vi "svc_Convert Frequency to Frequency String.vi"(7 "number of decimal places to add":i32, 10 "x-axis unit label":string="Hz", 11 "frequency [Hz]":dbl format="%.2f") -> (3 "frequency string":string)   [LabVIEW 2017]
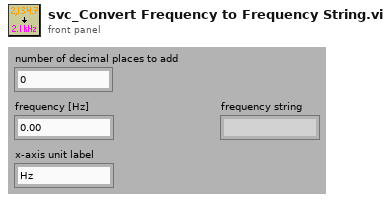
[diagram p1: front panel]
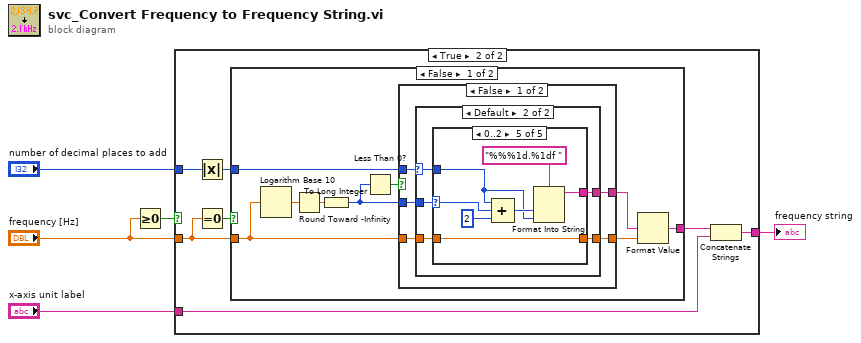
[diagram p0: block diagram]
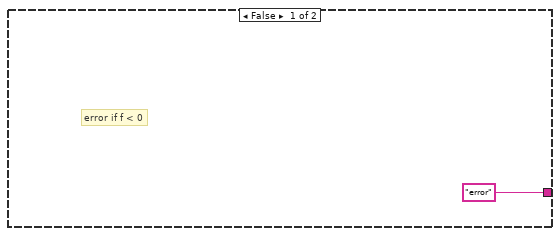
[diagram p2: hidden frame]
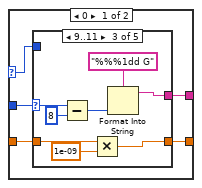
[diagram p3: hidden frame]
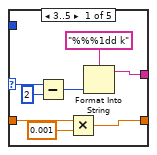
[diagram p4: hidden frame]
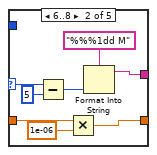
[diagram p5: hidden frame]
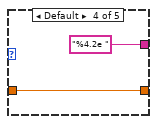
[diagram p6: hidden frame]
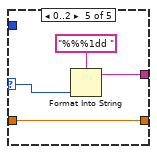
[diagram p7: hidden frame]
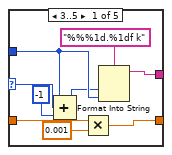
[diagram p8: hidden frame]
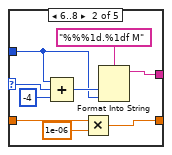
[diagram p9: hidden frame]
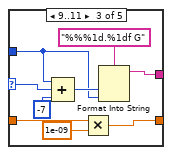
[diagram p10: hidden frame]
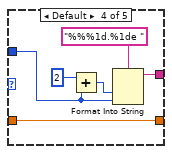
[diagram p11: hidden frame]
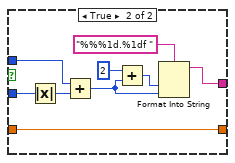
[diagram p12: hidden frame]
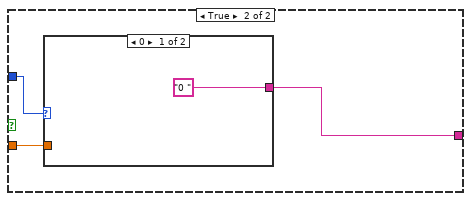
[diagram p13: hidden frame]
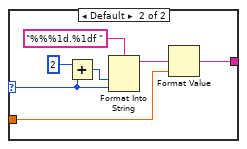
[diagram p14: hidden frame]
diagram:
  n1 = Greater Or Equal To 0?(x="frequency [Hz]") -> (x >= 0?=w3:bool)
  n2 = case shown="True" w3 {
    tunnel: ["error" ("output string") w9] -> w5
    tunnel: "frequency [Hz]" -> [_ w12]
    tunnel: "number of decimal places to add" -> [_ w11]
    tunnel: "x-axis unit label" -> [_ w7]
    frame False {
      # "error if f < 0"
    }
    frame True {
      n3 = Absolute Value(x=w11) -> (abs(x)=w10:i32)
      n4 = Equal To 0?(x=w12) -> (x = 0?=w13:bool)
      n5 = case shown="False" w13 {
        tunnel: [w22 w117] -> w8
        tunnel: w12 -> [w16 w118]
        tunnel: w10 -> [w14 w119]
        frame False {
          n6 = Logarithm Base 10(1:w16) -> (0:w17:dbl)
          n7 = Round Toward -Infinity ("Round To -Infinity")(1:w17) -> (0:w21:dbl)
          n8 = To Long Integer(number=w21) -> (32bit integer=w19:i32)
          n9 = Less Than 0?(x=w19) -> (x < 0?=w20:bool)
          n10 = case shown="False" w20 {
            tunnel: w19 -> [w27 w114]
            tunnel: [w26 w112] -> w18
            tunnel: w16 -> [w25 w111]
            tunnel: [w24 w111] -> w15
            tunnel: w14 -> [w23 w109]
            frame False {
              n11 = case shown="Default" w23 {
                selector: w23 -> [w31 w63]
                tunnel: w27 -> [w32 w67]
                tunnel: [w29 w66] -> w26
                tunnel: w25 -> [w30 w65]
                tunnel: [w28 w64] -> w24
                frame 0 {
                  n12 = case shown="9..11" w32 {
                    selector: w32 -> [w36 w44 w52 _ w59]
                    tunnel: [w34 w42 w50 "%4.2e " ("format string") w60] -> w29
                    tunnel: w30 -> [w40 w48 w56 w58 w62]
                    tunnel: [w38 w46 w54 w58 w62] -> w28
                    tunnel: w31 -> [_ _ _ _ _]
                    frame 3..5 {
                      n13 = Subtract(x=w36, y=2) -> (x-y=w37:i32)
                      n14 = Multiply(x=w40, y=0.001) -> (x*y=w38:dbl)
                      n15 = Format Into String(format string="%%%1dd k", w37) -> (resulting string=w34:string)  [unwired: 2 in, 1 out]
                    }
                    frame 6..8 {
                      n16 = Subtract(x=w44, y=5) -> (x-y=w45:i32)
                      n17 = Multiply(x=w48, y=1e-06) -> (x*y=w46:dbl)
                      n18 = Format Into String(format string="%%%1dd M", w45) -> (resulting string=w42:string)  [unwired: 2 in, 1 out]
                    }
                    frame 9..11 {
                      n19 = Subtract(x=w52, y=8) -> (x-y=w53:i32)
                      n20 = Multiply(x=w56, y=1e-09) -> (x*y=w54:dbl)
                      n21 = Format Into String(format string="%%%1dd G", w53) -> (resulting string=w50:string)  [unwired: 2 in, 1 out]
                    }
                    frame Default {
                    }
                    frame 0..2 {
                      n22 = Format Into String(format string="%%%1dd ", w59) -> (resulting string=w60:string)  [unwired: 2 in, 1 out]
                    }
                  }
                }
                frame Default {
                  n23 = case shown="0..2" w67 {
                    selector: w67 -> [w71 w82 w91 _ w106]
                    tunnel: [w73 w81 w90 w97 w101] -> w66
                    tunnel: w65 -> [w76 w85 w94 w100 w107]
                    tunnel: [w74 w83 w92 w100 w107] -> w64
                    tunnel: w63 -> [w70 w79 w87 w98 w103]
                    frame 3..5 {
                      n24 = Compound Arithmetic op=ADD(w70, w71, -1 ("y")) -> (w69:i32)
                      n25 = Multiply(x=w76, y=0.001) -> (x*y=w74:dbl)
                      n26 = Format Into String(format string="%%%1d.%1df k", w69, w70) -> (resulting string=w73:string)  [unwired: 2 in, 1 out]
                    }
                    frame 6..8 {
                      n27 = Compound Arithmetic op=ADD(w79, w82, -4 ("value")) -> (w80:i32)
                      n28 = Multiply(x=w85, y=1e-06) -> (x*y=w83:dbl)
                      n29 = Format Into String(format string="%%%1d.%1df M", w80, w79) -> (resulting string=w81:string)  [unwired: 2 in, 1 out]
                    }
                    frame 9..11 {
                      n30 = Compound Arithmetic op=ADD(w87, w91, -7 ("value")) -> (w88:i32)
                      n31 = Multiply(x=w94, y=1e-09) -> (x*y=w92:dbl)
                      n32 = Format Into String(format string="%%%1d.%1df G", w88, w87) -> (resulting string=w90:string)  [unwired: 2 in, 1 out]
                    }
                    frame Default {
                      n33 = Add(x=2 ("y"), y=w98) -> (x+y=w96:i32)
                      n34 = Format Into String(format string="%%%1d.%1de ", w96, w98) -> (resulting string=w97:string)  [unwired: 2 in, 1 out]
                    }
                    frame 0..2 {
                      n35 = Compound Arithmetic op=ADD(w103, w106, 2 ("value")) -> (w104:i32)
                      n36 = Format Into String(format string="%%%1d.%1df ", w104, w103) -> (resulting string=w101:string)  [unwired: 2 in, 1 out]
                    }
                  }
                }
              }
            }
            frame True {
              n37 = Absolute Value(x=w114) -> (abs(x)=w110:i32)
              n38 = Add(x=w109, y=w110) -> (x+y=w108:i32)
              n39 = Add(x=2 ("y"), y=w108) -> (x+y=w113:i32)
              n40 = Format Into String(format string="%%%1d.%1df ", w113, w108) -> (resulting string=w112:string)  [unwired: 2 in, 1 out]
            }
          }
          n41 = Format Value(format string=w18, value (0)=w15) -> (output string=w22:string)  [unwired: 1 in]
        }
        frame True {
          n42 = case shown="0" w119 {
            selector: w119 -> [_ w124]
            tunnel: ["0 " w121] -> w117
            tunnel: w118 -> [_ w122]
            frame 0 {
            }
            frame Default {
              n43 = Add(x=2 ("y"), y=w124) -> (x+y=w125:i32)
              n44 = Format Into String(format string="%%%1d.%1df ", w125, w124) -> (resulting string=w123:string)  [unwired: 2 in, 1 out]
              n45 = Format Value(format string=w123, value (0)=w122) -> (output string=w121:string)  [unwired: 1 in]
            }
          }
        }
      }
      n46 = Concatenate Strings(w8, w7) -> (w9:string)
    }
  }
  "frequency string" <- w5
